vi "UpdateWorld.vi"(8 "error in (no error)":errorcluster, 10 "World in":refnum<class "3D Object.lvclass">, 11 "Render Window in":refnum<class "Render Window.lvclass">) -> (0 "error out":errorcluster, 3 "Render Window out":refnum<class "Render Window.lvclass">)   [LabVIEW 2015, in "Render Window.lvclass"]
uses:
  Render Window.lvclass
  3D Object/3D Object.lvclass
  3D Object/3D Object.lvclass/3D Object.ctl
  Render Window.lvclass/Render Window.ctl
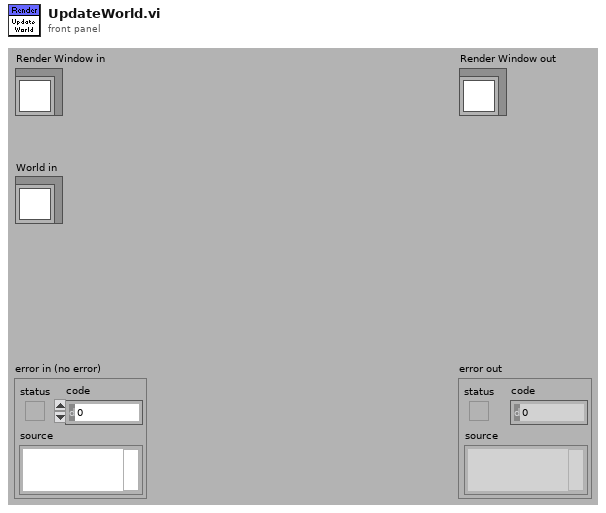
[diagram p1: front panel]
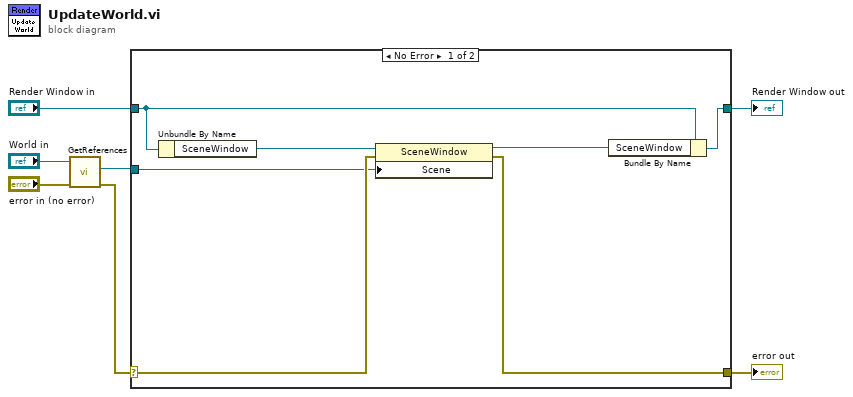
[diagram p0: block diagram]
diagram:
  n1 = call "GetReferences.vi"("error in (no error)"="error in (no error)", "3D Object in"="World in") -> ("error out"=w4:errorcluster, "SceneObject"=w1:refnum<vi>)  [unwired: 6 in, 2 out]
  n2 = case shown="No Error" w4 {
    selector: w4 -> [w9 w16]
    tunnel: [w11 w16] -> w7
    tunnel: [w12 w15] -> w5
    tunnel: "Render Window in" -> [w14 w15]
    tunnel: w1 -> [w8 _]
    frame No Error {
      n3 = Unbundle By Name(w14) -> ("SceneWindow"=w10:refnum<vi>)
      n4 = property class="SceneWindow"(reference=w10, error in=w9, "Scene"=w8) -> (reference out=w13:refnum<vi>, error out=w11:errorcluster)
      n5 = Bundle By Name(cluster=w14, "SceneWindow"=w13) -> (w12:refnum<class "Render Window.lvclass">)
    }
    frame Error {
    }
  }
  "error out" <- w7
  "Render Window out" <- w5
